vi "Test Black Board.vi"() -> ()   [LabVIEW 2021]
uses:
  Source/Blackboard/Blackboard.lvclass
  <vilib>/TSA/Abstract Data Classes/Abs_Types/Boolean/Static Write.vi
  <vilib>/TSA/Abstract Data Classes/Abs_Types/Boolean/Static Read.vi
  Source/Blackboard/Support/Bool/Blackboard_Boolean.lvclass
  C:/Program Files (x86)/National Instruments/LabVIEW 2021/vi.lib/TSA/Abstract Data Classes/Abs_Types/Boolean/Abs_Boolean.lvclass
  <vilib>/TSA/Abstract Data Classes/Abs_Types/Boolean/Abs_Boolean.lvclass
  C:/Program Files (x86)/National Instruments/LabVIEW 2021/vi.lib/TSA/Abstract Data Classes/Abs_Types/Value/Abs_Value.lvclass
  C:/Program Files (x86)/National Instruments/LabVIEW 2021/vi.lib/TSA/Abstract Data Classes/Abs_Types/Type/Abs_Type.lvclass
  C:/Users/Tim/Documents/GitHub/LV_Behaviour_Tree/Source/Blackboard/Support/Bool/Blackboard_Boolean.lvclass
panel:
  in  "Boolean 6":bool
  out "Boolean 5":bool
  in  "Boolean 4":bool
  out "Boolean 3":bool
  in  "stop":bool
  out "Boolean 2":bool
  in  "Boolean":bool
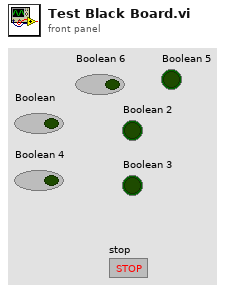
[diagram p1: front panel]
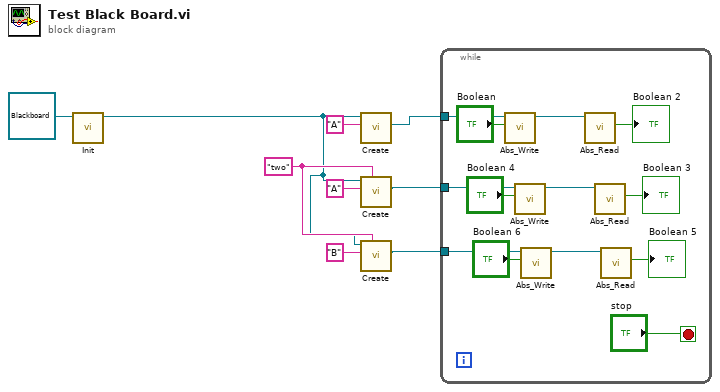
[diagram p0: block diagram]
diagram:
  w3 = "two" ("Group")
  n1 = call-dynamic "Init.vi"("bt_Blackboard in"=refnum<class "Blackboard.lvclass"> refnum) -> ("bt_Blackboard out"=w1:refnum<class "Blackboard.lvclass">)  [unwired: 9 in, 1 out]
  n2 = call "Create.vi"("Tag"="A", "Blackboard"=w1) -> ("Blackboard_Boolean.lvclass"=w7:refnum<class "Blackboard_Boolean.lvclass">)  [unwired: 7 in, 2 out]
  n3 = call "Create.vi"("Group"=w3, "Tag"="A", "Blackboard"=w1) -> ("Blackboard_Boolean.lvclass"=w5:refnum<class "Blackboard_Boolean.lvclass">)  [unwired: 6 in, 2 out]
  n4 = call "Create.vi"("Group"=w3, "Tag"="B", "Blackboard"=w1) -> ("Blackboard_Boolean.lvclass"=w2:refnum<class "Blackboard_Boolean.lvclass">)  [unwired: 6 in, 2 out]
  n5 = while {
    tunnel: w7 -> [w22]
    tunnel: w5 -> [w14]
    tunnel: w2 -> [w10]
    stop <- "stop" stop-if-true
    n6 = call-poly <vilib>:"Abs_Write.vi"("Boolean"="Boolean", "Abs_Boolean in"=w22) -> ("Abs_Boolean out"=w20:refnum<class "Blackboard_Boolean.lvclass">)  [unwired: 8 in, 1 out]
    n7 = call-poly <vilib>:"Abs_Write.vi"("Boolean"="Boolean 4", "Abs_Boolean in"=w14) -> ("Abs_Boolean out"=w16:refnum<class "Blackboard_Boolean.lvclass">)  [unwired: 8 in, 1 out]
    n8 = call-poly <vilib>:"Abs_Write.vi"("Boolean"="Boolean 6", "Abs_Boolean in"=w10) -> ("Abs_Boolean out"=w12:refnum<class "Blackboard_Boolean.lvclass">)  [unwired: 8 in, 1 out]
    n9 = call-poly <vilib>:"Abs_Read.vi"("Abs_Boolean in"=w20) -> ("Boolean"=→"Boolean 2":bool)  [unwired: 8 in, 2 out]
    n10 = call-poly <vilib>:"Abs_Read.vi"("Abs_Boolean in"=w16) -> ("Boolean"=→"Boolean 3":bool)  [unwired: 8 in, 2 out]
    n11 = call-poly <vilib>:"Abs_Read.vi"("Abs_Boolean in"=w12) -> ("Boolean"=→"Boolean 5":bool)  [unwired: 8 in, 2 out]
  }
